vi "ParseVectorFile.SVG.ImageFactory.vi"(8 "error in (no error)":errorcluster, 11 "ParseVectorFile in":refnum<class "ParseVectorFile.lvclass">) -> (0 "error out":errorcluster, 3 "ParseVectorFile out":refnum<class "ParseVectorFile.lvclass">)   [LabVIEW 2019, in "ParseVectorFile.lvclass"]
uses:
  ParseVectorFile.lvclass
  ParseVectorFile.lvclass/ParseVectorFile.ctl
  ParseXML/ParseSVG.lvclass/ParseSVG.ctl
  Image/SVGImage.lvclass
  Image/InitializationInfo.ctl
  ParseXML/ParseSVG.lvclass
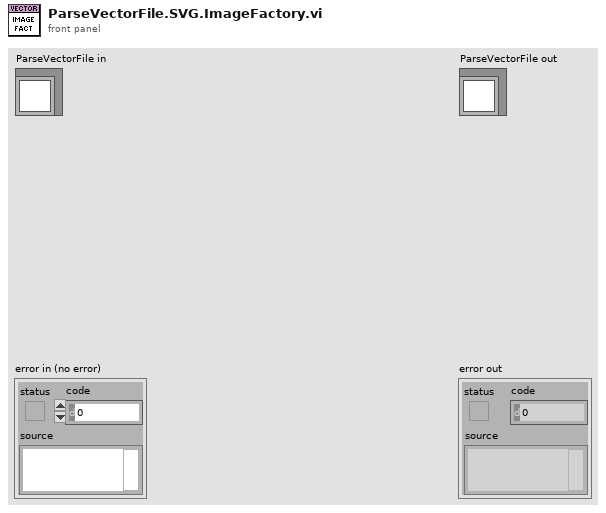
[diagram p1: front panel]
types:
  T1 = typedef "ParseSVG.lvclass/Image.ctl" = cluster{"x":string, "y":string, "width":string, "height":string, "xlink:href":string, "id":string}
  T2 = typedef "SVGImage.lvclass/InitializationInfo.ctl" = cluster{"X":string, "Y":string, "Width":string, "Height":string, "File Path":string, "ID":string}
  T3 = cluster{"Node Name":string, "Node SVG ID":string, "Attribute Name":string, "New Attribute Value":string}
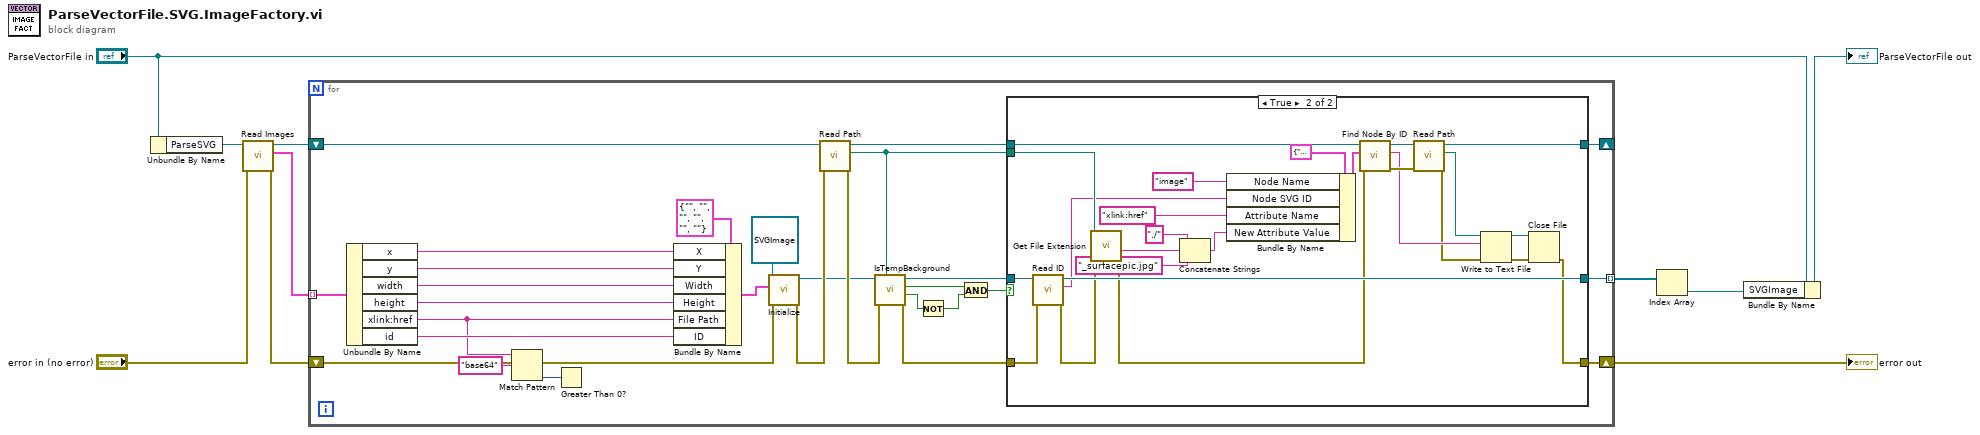
[diagram p0: block diagram]
diagram:
  n1 = Unbundle By Name("ParseVectorFile in") -> ("ParseSVG"=w5:refnum<class "ParseSVG.lvclass">)
  n2 = call "Read Images.vi"("error in (no error)"="error in (no error)", "ParseSVG in"=w5) -> ("error out"=w8:errorcluster, "Images"=w4:T1[], "ParseSVG out"=w1:refnum<class "ParseSVG.lvclass">)  [unwired: 7 in]
  n3 = for {
    tunnel: [w24] -> w3 mode=indexing
    shift-right: [w27] -> w7
    shift-left: w8 -> [w31]
    tunnel: w4 -> [w29] mode=indexing
    shift-right: [w28] -> _
    shift-left: w1 -> [w19]
    n4 = Unbundle By Name(w29) -> ("x"=w37:string, "y"=w36:string, "width"=w35:string, "height"=w34:string, "xlink:href"=w13:string, "id"=w30:string)
    n5 = Match Pattern(string=w13, regular expression="base64") -> (offset past match=w11:i32)  [unwired: 1 in, 3 out]
    n6 = Greater Than 0?(x=w11) -> ()  [unwired: 1 out]
    n7 = Bundle By Name(cluster=T2 {"X"="", "Y"="", "Width"="", "Height"="", "File Path"="", "ID"=""} ("Info"), "X"=w37, "Y"=w36, "Width"=w35, "Height"=w34, "File Path"=w13, "ID"=w30) -> (w33:T2)
    n8 = call "Initialize.vi"("error in (no error)"=w31, "Info"=w33, "Image in"=refnum<class "SVGImage.lvclass"> refnum) -> ("error out"=w17:errorcluster, "Image out"=w15:refnum<class "SVGImage.lvclass">)  [unwired: 7 in]
    n9 = call-dynamic "Read Path.vi"("error in (no error)"=w17, "ParseSVG in"=w19) -> ("error out"=w16:errorcluster, "Path"=w14:path, "ParseSVG out"=w18:refnum<class "ParseSVG.lvclass">)  [unwired: 7 in]
    n10 = call "IsTempBackground.vi"("SVG Path"=w14, "error in"=w16, "SVGImage in"=w15) -> ("error out"=w25:errorcluster, "Correct Location"=w22:bool, "Is background?"=w23:bool, "SVGImage out"=w26:refnum<class "SVGImage.lvclass">)  [unwired: 5 in]
    n11 = Not(x=w22) -> (.not. x?=w21:bool)
    n12 = And(x=w23, y=w21) -> (x .and. y?=w20:bool)
    n13 = case shown="True" w20 {
      tunnel: w18 -> [w41 w66]
      tunnel: [w41 w58] -> w28
      tunnel: [w39 w51] -> w27
      tunnel: w26 -> [w40 w65]
      tunnel: w25 -> [w39 w64]
      tunnel: [w40 w63] -> w24
      tunnel: w14 -> [_ w47]
      frame False {
      }
      frame True {
        n14 = call-dynamic "Read ID.vi"("error in (no error)"=w64, "SVGImage in"=w65) -> ("error out"=w50:errorcluster, "ID"=w44:string, "SVGImage out"=w63:refnum<class "SVGImage.lvclass">)  [unwired: 7 in]
        n15 = call <vilib>:"Get File Extension.vi"("error in (no error)"=w50, "file"=w47) -> ("error out"=w49:errorcluster, "filename without extension"=w48:string)  [unwired: 5 in, 3 out]
        n16 = Concatenate Strings("./" ("string"), w48, "_surfacepic.jpg" ("string")) -> (w45:string)
        n17 = Bundle By Name(cluster=T3 {"Node Name"="", "Node SVG ID"="", "Attribute Name"="", "New Attribute Value"=""} ("Node Info"), "Node Name"="image" ("Node Name (exact)"), "Node SVG ID"=w44, "Attribute Name"="xlink:href", "New Attribute Value"=w45) -> (w60:T3)
        n18 = call "Find Node By ID.vi"("error in (no error)"=w49, "Node Info"=w60, "ParseSVG in"=w66) -> ("error out"=w57:errorcluster, "Corrected XML"=w56:string, "ParseSVG out"=w59:refnum<class "ParseSVG.lvclass">)  [unwired: 6 in]
        n19 = call-dynamic "Read Path.vi"("error in (no error)"=w57, "ParseSVG in"=w59) -> ("error out"=w54:errorcluster, "Path"=w55:path, "ParseSVG out"=w58:refnum<class "ParseSVG.lvclass">)  [unwired: 7 in]
        n20 = Write to Text File(file (use dialog)=w55, text=w56, error in=w54) -> (refnum out=w53:refnum<file>, error out=w52:errorcluster)  [unwired: 1 in, 1 out]
        n21 = Close File(refnum=w53, error in=w52) -> (error out=w51:errorcluster)  [unwired: 1 out]
      }
    }
  }
  "error out" <- w7
  n22 = Index Array(array=w3) -> (element=w2:refnum<class "SVGImage.lvclass">)  [unwired: 1 in]
  n23 = Bundle By Name(cluster="ParseVectorFile in", "SVGImage"=w2) -> (→"ParseVectorFile out":refnum<class "ParseVectorFile.lvclass">)
